vi "Bar.vi"() -> (1 "Time Out Value":u8, 2 "Barcode Scane":bool, 3 "Out":bool)   [LabVIEW 2015]
uses:
  Control Button/Exit.ctl
  Feature list/Control PB/Next_.ctl
panel:
  in  "Time Out (ms)":u8
  in  "Barcode":bool
  in  "Next":T1
  in  "Exit":T2
  # "Add Feature List"
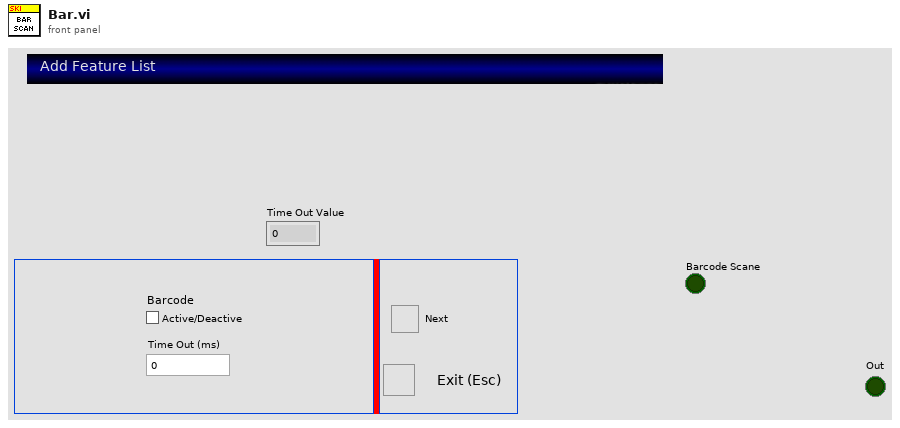
[diagram p1: front panel]
types:
  T1 = typedef "Next_.ctl" = bool
  T2 = typedef "Exit.ctl" = bool
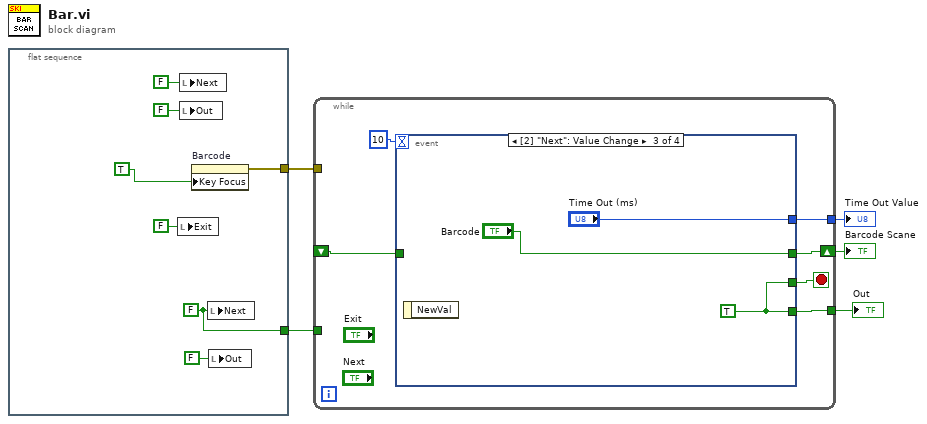
[diagram p0: block diagram]
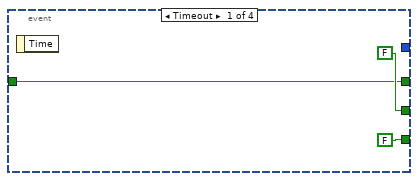
[diagram p2: hidden frame]
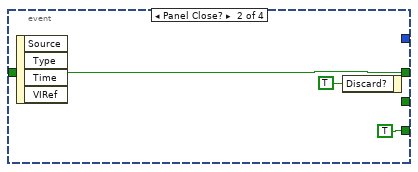
[diagram p3: hidden frame]
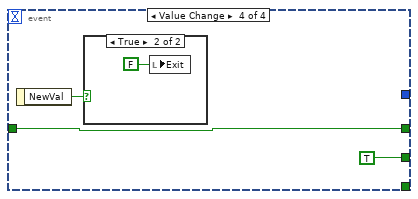
[diagram p4: hidden frame]
diagram:
  n1 = flat-sequence {
    tunnel: [w9] -> w4
    tunnel: [w6] -> w3
    frame #0 {
      w9 = T1 FALSE ("Next")
      n2 = local write "Exit"(FALSE ("Exit")) -> ()
      n3 = local write "Next"(T1 FALSE ("Next")) -> ()
      n4 = local write "Out"(FALSE ("Out")) -> ()
      n5 = property on="Barcode" class="Bool (strict)"("Key Focus"=TRUE) -> (error out=w6:errorcluster)  [unwired: 2 in, 1 out]
      n6 = local write "Next"(w9) -> ()
      n7 = local write "Out"(FALSE ("Out")) -> ()
    }
  }
  n8 = while {
    tunnel: [w16] -> w5
    tunnel: w4 -> [_]
    shift-right: [w17] -> w2
    shift-left: _ -> [w14]
    tunnel: w3 -> [_]
    tunnel: [w13] -> w1
    stop <- w18 stop-if-true
    n9 = event shown="[2] \"Next\": Value Change" {
      selector: _ -> [_ _ _ _]
      dyn-events: _ -> [_ _ _ _]
      timeout: 10 -> [_ _ _ _]
      tunnel: [FALSE _ w26 TRUE] -> w18
      tunnel: [w19 w22 "Barcode" w28] -> w17
      tunnel: [T1 FALSE ("NewVal") T1 TRUE ("NewVal") w26 _] -> w16
      tunnel: w14 -> [w19 w22 _ w28]
      tunnel: [_ _ "Time Out (ms)" _] -> w13
      event Timeout {
        n10 = event-data() -> ()  [unwired: 1 in, 1 out]
      }
      event Panel Close? {
        n11 = event-data() -> ()  [unwired: 1 in, 4 out]
        n12 = event-data("Discard?"=TRUE) -> ()  [unwired: 1 in, 1 out]
      }
      event Value Change {
        w26 = T1 TRUE ("NewVal")
        n13 = event-data() -> ()  [unwired: 1 in, 1 out]
      }
      event Value Change {
        n14 = event-data() -> ("NewVal"=w29:T2)  [unwired: 1 in]
        n15 = case shown="True" w29 {
          frame False {
          }
          frame True {
            n16 = local write "Exit"(T1 FALSE ("Next")) -> ()
          }
        }
      }
    }
  }
  "Out" <- w5
  "Barcode Scane" <- w2
  "Time Out Value" <- w1
